vi "Global Read.vi"(8 "error in (no error)":errorcluster, 11 "Pump Number":i32) -> (0 "error out":errorcluster, 1 "ChannelCnt":dbl, 2 "Initialized":bool, 3 "Busy":bool, 4 "Current Channel":dbl, 5 "Ismatec 4083 Global":T1, 6 "Initialized Channels":dbl[](array[numeric]))   [LabVIEW 2018, in "Ismatec 4308.lvlib"]
uses:
  Ismatec 4308.lvlib
  Ismatec 4083 Global.ctl
  Ismatec 4083 Global Element.ctl
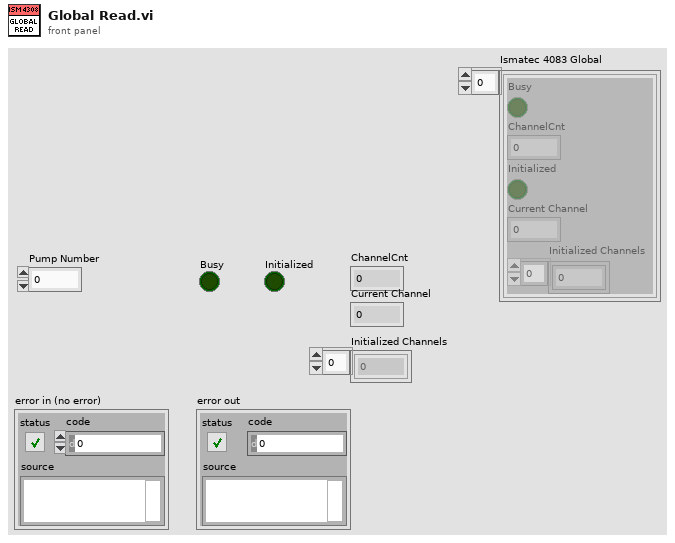
[diagram p1: front panel]
types:
  T1 = typedef "Ismatec 4308.lvlib/Ismatec 4083 Global.ctl" = T2[]
  T2 = typedef "Ismatec 4308.lvlib/Ismatec 4083 Global Element.ctl" = cluster{"Busy":bool, "ChannelCnt":dbl, "Initialized":bool, "Current Channel":dbl, "Initialized Channels":dbl[]}
  T3 = cluster{"Busy":bool, "ChannelCnt":dbl, "Initialized":bool, "Current Channel":dbl, "Initialized Channels":dbl[]}[]
  T4 = cluster{"Busy":bool, "ChannelCnt":dbl, "Initialized":bool, "Current Channel":dbl, "Initialized Channels":dbl[]}
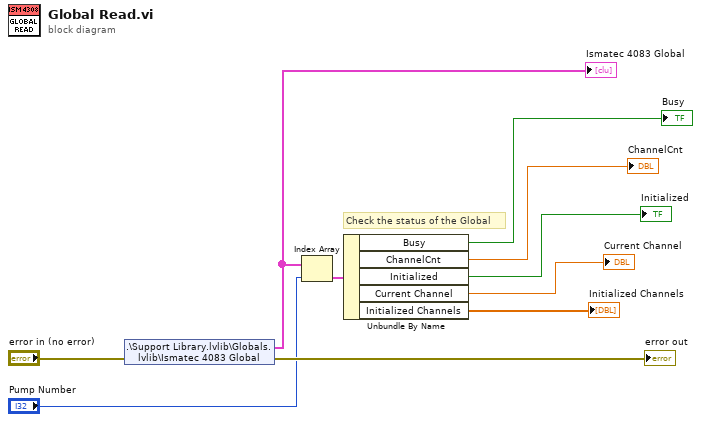
[diagram p0: block diagram]
diagram:
  # "Check the status of the Global"
  n1 = shared-variable ".\\Support Library.lvlib\\Globals.lvlib\\Ismatec 4083 Global"(error in="error in (no error)") -> (w3:T3, error out=→"error out":errorcluster)
  "Ismatec 4083 Global" <- w3
  n2 = Index Array(array=w3, index="Pump Number") -> (element=w7:T4)
  n3 = Unbundle By Name(w7) -> ("Busy"=→"Busy":bool, "ChannelCnt"=→"ChannelCnt":dbl, "Initialized"=→"Initialized":bool, "Current Channel"=→"Current Channel":dbl, "Initialized Channels"=→"Initialized Channels":dbl[])
